vi "SetOnCircle.vi"(7 "angle (deg)":dbl, 8 "error in (no error)":errorcluster, 9 "Radius":dbl, 10 "Center":T1, 11 "GameObject in":refnum<class "GameObject.lvclass">) -> (0 "error out":errorcluster, 3 "GameObject out":refnum<class "GameObject.lvclass">)   [LabVIEW 2019, in "RT_Game.lvlib" / "GameObject.lvclass"]
uses:
  GameObject.lvclass
  Game/Coordinate.ctl
  Game/Game.lvclass
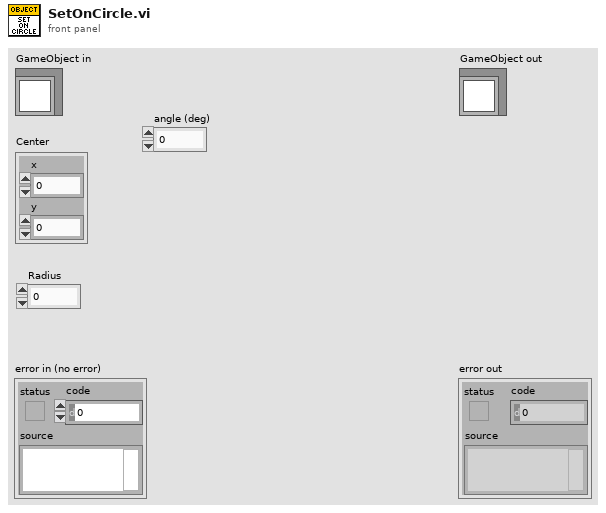
[diagram p1: front panel]
types:
  T1 = typedef "RT_Game.lvlib/Game.lvclass/Coordinate.ctl" = cluster{"x":dbl, "y":dbl}
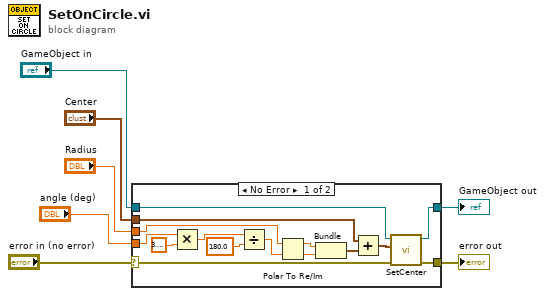
[diagram p0: block diagram]
diagram:
  n1 = case shown="No Error" "error in (no error)" {
    selector: "error in (no error)" -> [w9 w24]
    tunnel: [w8 w24] -> w6
    tunnel: [w10 w23] -> w1
    tunnel: "GameObject in" -> [w11 w23]
    tunnel: "Center" -> [w19 _]
    tunnel: "Radius" -> [w22 _]
    tunnel: "angle (deg)" -> [w15 _]
    frame No Error {
      n2 = Multiply(x=w15, y=3.141592653589793) -> (x*y=w14:dbl)
      n3 = Divide(x=w14, y=180.0) -> (x/y=w12:dbl)
      n4 = Polar To Re/Im(2:w12, 3:w22) -> (0:w20:dbl, 1:w21:dbl)
      n5 = Bundle(w21, w20) -> (w18:cluster{dbl, dbl})  [unwired: 1 in]
      n6 = Add(x=w19, y=w18) -> (x+y=w17:T1)
      n7 = call "SetCenter.vi"("error in (no error)"=w9, "center_position"=w17, "GameObject in"=w11) -> ("error out"=w8:errorcluster, "GameObject out"=w10:refnum<class "GameObject.lvclass">)  [unwired: 7 in]
    }
    frame Error {
    }
  }
  "error out" <- w6
  "GameObject out" <- w1
